vi "Get Needle Base.vi"(8 "error in (no error)":errorcluster, 11 "Item Ref in":T1 format="%.0x") -> (0 "error out":errorcluster, 2 "Needle Base":cluster{"X":sgl, "Y":sgl}, 3 "Item Ref out":T1 format="%.0x")   [LabVIEW 2011, in "Meter Detection Custom Device.lvlib"]
uses:
  Meter Detection Custom Device.lvlib
  <vilib>/NI Veristand/Custom Device API/Custom Device Item Ref.ctl
  Meter Detection Global Variable.vi
  <vilib>/NI Veristand/Custom Device API/Get Item Property (Variant).vi
  <vilib>/NI Veristand/Custom Device API/Custom Device API.lvlib
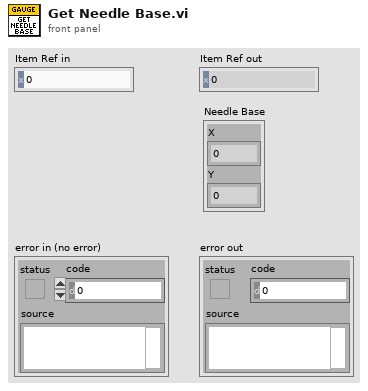
[diagram p1: front panel]
types:
  T1 = typedef "Custom Device API.lvlib/Custom Device Item Ref.ctl" = u64
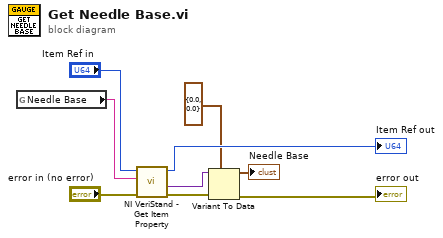
[diagram p0: block diagram]
diagram:
  n1 = global read "Meter Detection Global Variable.vi" "Needle Base"() -> (w8:string)
  n2 = call-poly <vilib>:"NI VeriStand - Get Item Property.vi"("error in (no error)"="error in (no error)", "Property Name"=w8, "Item Ref in"="Item Ref in") -> ("error out"=w5:errorcluster, "Value"=w4:variant, "Item Ref out"=→"Item Ref out":T1)  [unwired: 5 in, 1 out]
  n3 = Variant To Data(error in=w5, type=cluster{"X":sgl, "Y":sgl} {"X"=0.0, "Y"=0.0} ("Needle Base"), Variant=w4) -> (data=→"Needle Base":cluster{"X":sgl, "Y":sgl}, error out=→"error out":errorcluster)
